vi "BM_Detect_Integrate_Peaks.vi"(8 "stop":bool, 9 "Use as SubVI?":bool, 10 "Drop\npt.s?":i32=1, 11 "Imported Data":dbl[][](array[numeric])=array14000x8[112000 elements]) -> (2 "Peak Area":dbl=9488.210393014257 format="%#_4e", 3 "Peak Height":dbl=499.997845207867 format="%#_4e")   [LabVIEW 2021]
uses:
  <vilib>/Analysis/6fits.llb/Curve Fitting Criteria.ctl
  <vilib>/Utility/miscctls.llb/LVAnnotationListTypeDef.ctl
  <vilib>/Analysis/NI_AALPro.lvlib
  <vilib>/ptbypt/NI_PtbyPt.lvlib
  <vilib>/Analysis/NI_AAL_SigProc.lvlib
  <vilib>/Analysis/NI_AALBase.lvlib
panel:
  in  "Tab Control":enum32{"GUI", "Imported Raw Data"}(tab)
  in  "Reset Plots":bool
  in  "Analyte":u16(ring) items=["62 m/z", "63 m/z", "65 m/z", "68 m/z", "70 m/z"]
  out "Detection Limit":dbl=5.772939383333335 caption="LOD" format="%#_3g"
  out "Integrated Data":cluster{dbl[], dbl[]}(graph)
  out "Data":T1(graph)
  out "X Click Coordinates":dbl=462.027422648
  out "Y Click Coordinates":dbl=59.0625
  out "Closest X Data pt.":dbl=463.592079
  out "Closest Y Data pt.":dbl=59.95878535601133
  in  "Filename":path=path "C:/Users/bcamc/OneDrive/Desktop/2022_cruise_data/CIMS_Data/Brandon_CIMS_07102022_02.lvm"
  out "X Data":dbl[](array[numeric])
  out "Y Data":dbl[](array[numeric])
  in  "YData Index":i32=7
  out "Number of Points Selected":i32
  in  "XData Index":i32=6
  in  "Width":i32=6
  in  "Correct Baseline\nOrder":bool=TRUE
  in  "Apply Boxcar Filter":bool
  out "Filtered Y":dbl[](array[numeric])
  out "Baseline Corrected Y":dbl[](array[numeric])
  out "Boxcar Progress":u8(slide) scale=0.0..100.0
  in  "Autofix Y Scale":bool=TRUE
  out "Integral Y":dbl[](array[numeric])=[40.03240345107625, -9.96789609639881, -19.96819647164608, 10.03150332578528, 10.031203296894425, -29.96909656031754, 10.030604753152069, -19.96969475828041, 0.030005903961438207, -19.97029326311293, -9.970592257508663, -29.970890086087266, 10.028811265294742, 30.02851278935423, -9.97178650433171, -29.97208562617694, -19.97238259366285, 20.027319623664553, -9.972977989306159, 50.02672358284819, -19.973574669190057, 30.02612922441501, 20.025832303719383, -29.974464444298768, 20.025238980360562, 30.02494159358664, -19.97535562133391, -49.97565069453216, -9.975946577602919, -39.97624228898213, 0.023462172316150998, 0.02316582365677533, 0.022871612945145614, -19.977423409689074, -29.977718255715935, 0.021987068969757217, 10.021691586570974, -29.978601763626443, 20.02110407713249, -19.979189906491733, -29.979484695881453, 40.02022069149108, 20.01992820042487, -29.980365093871676, 20.01934081422818, 0.019046892249846792, -19.98124685394985, -9.981538482377943, 0.01816908786275917, 20.017876832728625, 50.01758474832545, 20.01729186740849, 30.017001099498053, 40.016709535071534, 20.016418140410195, 20.016126917458827, -29.984164126026975, 20.0155459640702, 30.015255262455305, 20.014964732549217, 30.01467437435368, 50.0143832263437, 30.01409417889586, 40.013804338734495, 20.013514671251755, 60.01322517741171, 70.01293489662064, 120.01264670776405, 40.012357731956456, 80.01206797091655, 80.01177838177952, 50.01148896454879, 80.01120164120061, 70.01091353088685, 90.01062559133166, 130.0103378234968, 170.01004927444615, 140.00976280969502, 190.00947556372347, 140.00918848755913, 190.00890158502887, 250.00861485326635, 270.0083292484607, 200.00804286338996, 260.0077566519498, 290.0074706112809, 310.00718379607423, 260.0068990498817, 250.0066135291492, 290.006328181093, 310.00604300191446, 250.00575799826413, 400.0054722225604, 270.0051885099438, 440.00490402432536, 350.0046197113844, 360.00433557017465, 290.00405065977725, 470.00376780768124, 350.0034841854507, 280.0032007368416, 380.0029165185042, 420.00263247493706, 310.00235048204814, 410.002067725663, 440.00178514007087, 290.00150272621573, 370.00122048691907, 320.0009393568023, 410.00065746040724, 300.00037480133426, 410.00009231702643, 379.9998100065449, 399.9995297371525, 429.9992487062318, 459.9989678470532, 359.9986862295762, 319.9984047849914, 439.99812537762523, 499.997845207867, 389.9975642849034, 369.9972844638737, 329.99700388798567, 239.99672534077752, 279.9964460377797, 339.9961669074594, 439.99588794981656, 309.99560823832314, 369.9953305516355, 329.995052112953, 419.9947738450934, 369.9944957499124, 349.9942178292611, 419.99394100252186, 359.99366342572597, 159.9933851005939, 199.99310694836495, 229.9928289718088, 179.99255300488858, 329.9922762926282, 249.9919997539662, 369.9917224676506, 229.991445357923, 169.99117025485873, 219.99089440564006, 199.99061873093612, 269.990343227991, 179.99006698268045, 209.98979274013325, 209.98951775338915, 189.9892429420703, 79.98896830159859, 179.9886938319775, 119.98842045120503, 69.9881463300203, 249.98787237877505, 139.9875986029447, 149.98732499979067, 109.98705065967226, 139.98677827602253, 139.986505222749, 209.98623140329462, 49.9859577558501, 129.9856842840496, 179.9854127957304, 69.98514057423267, 79.98486762127854, 129.98459484396267, 119.98432223956722, 109.98405161019505, 79.98378025323284, 129.98350906894808, 119.98323805824333, 59.982966318299475, 129.98269655125742, 149.98242605858394, 119.98215573768661, 99.98188558856715, 39.98161561482343, 159.98134670683015, 169.98107707606925, 99.98080761888315, 69.9805383325799, 29.98026832458241, 39.98000027890487, 69.97973151332198, 49.97946291773094, 69.97919360274193, 99.97892446515473, 69.97865727788658, 59.97838937447513, -0.0218783562588456, 39.97785408746663, 39.97758670030564, 39.97732037477243, 89.97705333328562, 109.97678646714353, 19.97651977190037, 99.97625324844716, 89.97598778374929, 69.9757216050787, 49.975455600858375, 69.97518888496157, 49.974922343776946, 69.97465773751549, 59.974392425460934, 19.974127284315678, 59.97386143613493, 89.97359576178053, 49.97333201661638, 39.97306756763633, 89.9728032913326, 9.972539185946232, 59.97227437608945, -30.02798850503394, 29.971747907614443, 79.97148449469582, 79.9712212527003, 89.97095818338343, 9.970696161327204, -0.02956656145727976, 19.97017088756025, 79.96990850838154, 79.9696463027546, 29.969383399841476, 39.969122410405184, 19.968860721938682, -10.031400792978324, 69.96833699624216, 29.968074959290135, 19.967814830074538, -10.032445993557914, 49.96729248924528, -0.03296885238920311, 29.966769978067866, 39.96651071138221, 9.966250752284147, 49.965990965863554, 129.96573048846227, -10.034529811654537, 59.965211780157794, 19.96495268674736, 29.964693763425437, 49.96443501450545, -20.03582356259929, 29.96391889088816, -0.03633934229502245, 39.963402598919124, 19.96314471109205, 19.962886139464665, 89.96262945433142, -10.037627913746242, 39.96211488999596, 19.961857865559736, 9.961600162759488, 69.96134433728743, -0.03891216826045252, 29.96083064698272, 29.960573636053397, 9.960316799804033, 19.960061835996257, -0.040193805016087936, 79.95955072579832, -40.04070456900835, 9.959039460147565, 59.95878535601133]
  in  "polynomial order":i32=2
  in  "Threshold":dbl=650.0 format="%0.2f"
  in  "Width":i32=25 min=3
  out "Peaks\nFound":i32
  in  "Auto Detect Peaks":bool=TRUE
  out "n Blanks":i32
  in  "Calculate LOD":bool caption="2. Add Std. Peak"
  in  "Add Next Blank":bool caption="1. Add Blank Peaks (³3)"
  in  "Std. Conc.":dbl
  out "Peak Start Time":string="00:06:24"
  out "Peak Height Time":string="00:06:60"
  in  "Imported Data Table":string[][](table)=array14000x8[112000 elements]
  out "Peak \nLocations (mins)":dbl[](array[numeric])
  out "Peak \nAmplitudes":dbl[](array[numeric])
  out "Retention\nTime (min)":dbl[](array[numeric])
  out "Mean Retention Time (Min)":dbl format="%#_3g"
  # "Find and Integrate Peaks"
  # "Select Data"
  # "Selected Data Points"
  # "Integrated Peak"
  # "nM"
  # "nM"
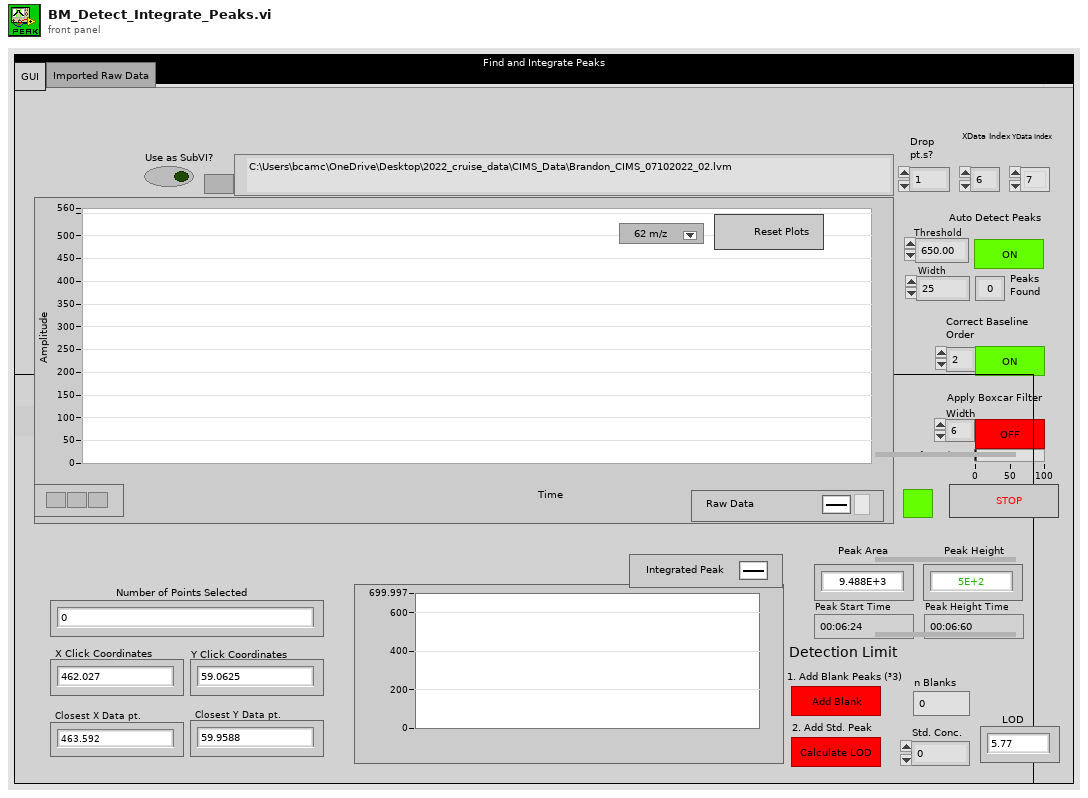
[diagram p1: front panel]
types:
  T1 = cluster{"Integral X Data":dbl[], "Integral Y Data":dbl[]}[]
  T2 = typedef "LVAnnotationListTypeDef.ctl" = cluster{"Name":string, "Color":u32, "Style":u8, "Point Style":u8, "Name Visible":bool, "Allow Drag":bool, "Annotation Mode":u32, "Plot":i32, "Index":i32, "Position":cluster{"X":dbl, "Y":dbl}, "X Scale":u32, "Y Scale":u32, "Show Arrow":bool, "Lock Name":bool, "Plot Area":i32, "Label Offset":cluster{"X":dbl, "Y":dbl}}[]
  T3 = typedef "NI_AALPro.lvlib/Curve Fitting Criteria.ctl" = u16
  T4 = cluster{"Integral X Data":dbl[], "Integral Y Data":dbl[]}
  T5 = cluster{"Name":string, "Color":u32, "Style":u8, "Point Style":u8, "Name Visible":bool, "Allow Drag":bool, "Annotation Mode":u32, "Plot":i32, "Index":i32, "Position":cluster{"X":dbl, "Y":dbl}, "X Scale":u32, "Y Scale":u32, "Show Arrow":bool, "Lock Name":bool, "Plot Area":i32, "Label Offset":cluster{"X":dbl, "Y":dbl}}
  T6 = cluster{"X Data":dbl[], "Baseline Corrected Y":dbl[]}
  T7 = typedef "LVPoint32TypeDef.ctl" = cluster{"Horizontal":i32, "Vertical":i32}
  T8 = typedef "LVRectTypeDef.ctl" = cluster{"Left":i16, "Top":i16, "Right":i16, "Bottom":i16}
  T9 = cluster{string, u32, i32, i32, bool, bool, i32, i32, i32, cluster{dbl, dbl}}
  T10 = cluster{string, u32, i32, i32, bool, bool, i32, i32, i32, cluster{dbl, dbl}}[]
  T11 = cluster{"Name":string, "Color":u32, "Style":u8, "Point Style":u8, "Name Visible":bool, "Allow Drag":bool, "Annotation Mode":u32, "Plot":i32, "Index":i32, "Position":cluster{"X":dbl, "Y":dbl}, "X Scale":u32, "Y Scale":u32, "Show Arrow":bool, "Lock Name":bool, "Plot Area":i32, "Label Offset":cluster{"X":dbl, "Y":dbl}}[]
  T12 = cluster{"X Data":dbl[], "Baseline Corrected Y":dbl[]}[]
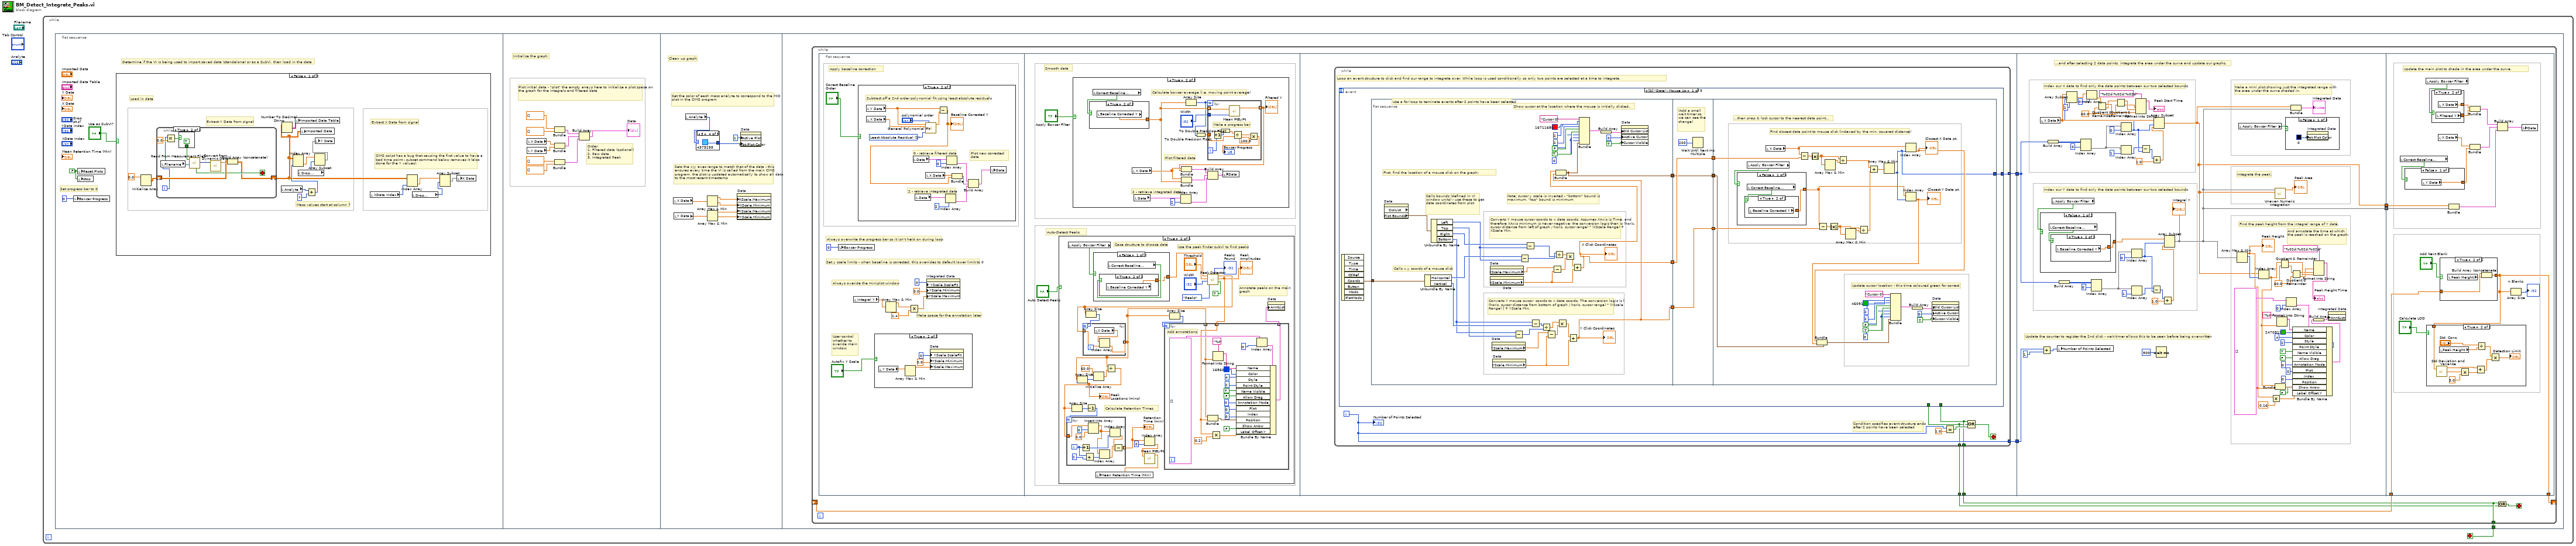
[diagram p0: block diagram]
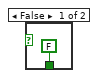
[diagram p2: hidden frame]
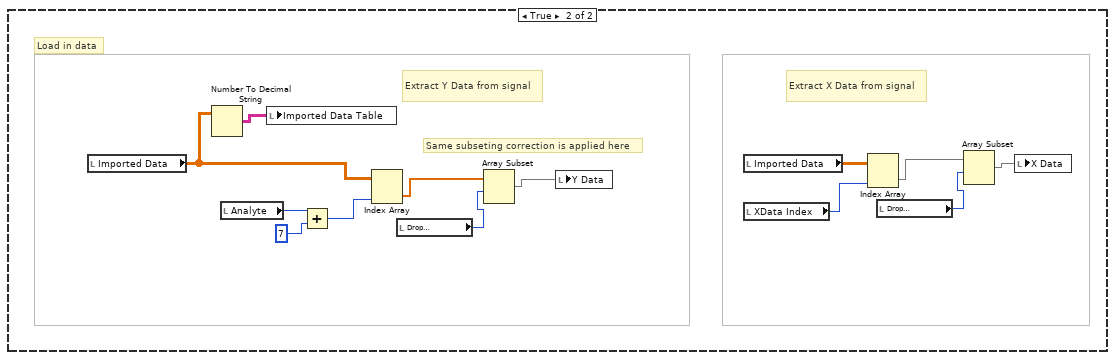
[diagram p3: hidden frame]
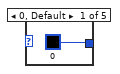
[diagram p4: hidden frame]
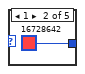
[diagram p5: hidden frame]
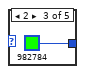
[diagram p6: hidden frame]
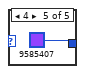
[diagram p7: hidden frame]
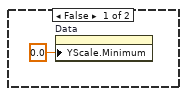
[diagram p8: hidden frame]
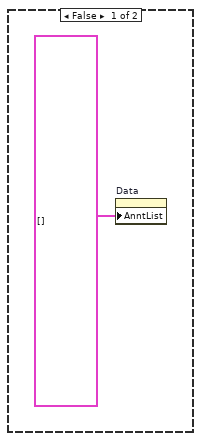
[diagram p10: hidden frame]
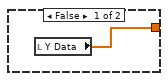
[diagram p11: hidden frame]
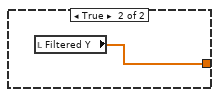
[diagram p12: hidden frame]
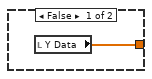
[diagram p14: hidden frame]
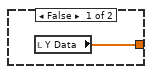
[diagram p15: hidden frame]
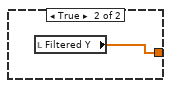
[diagram p16: hidden frame]
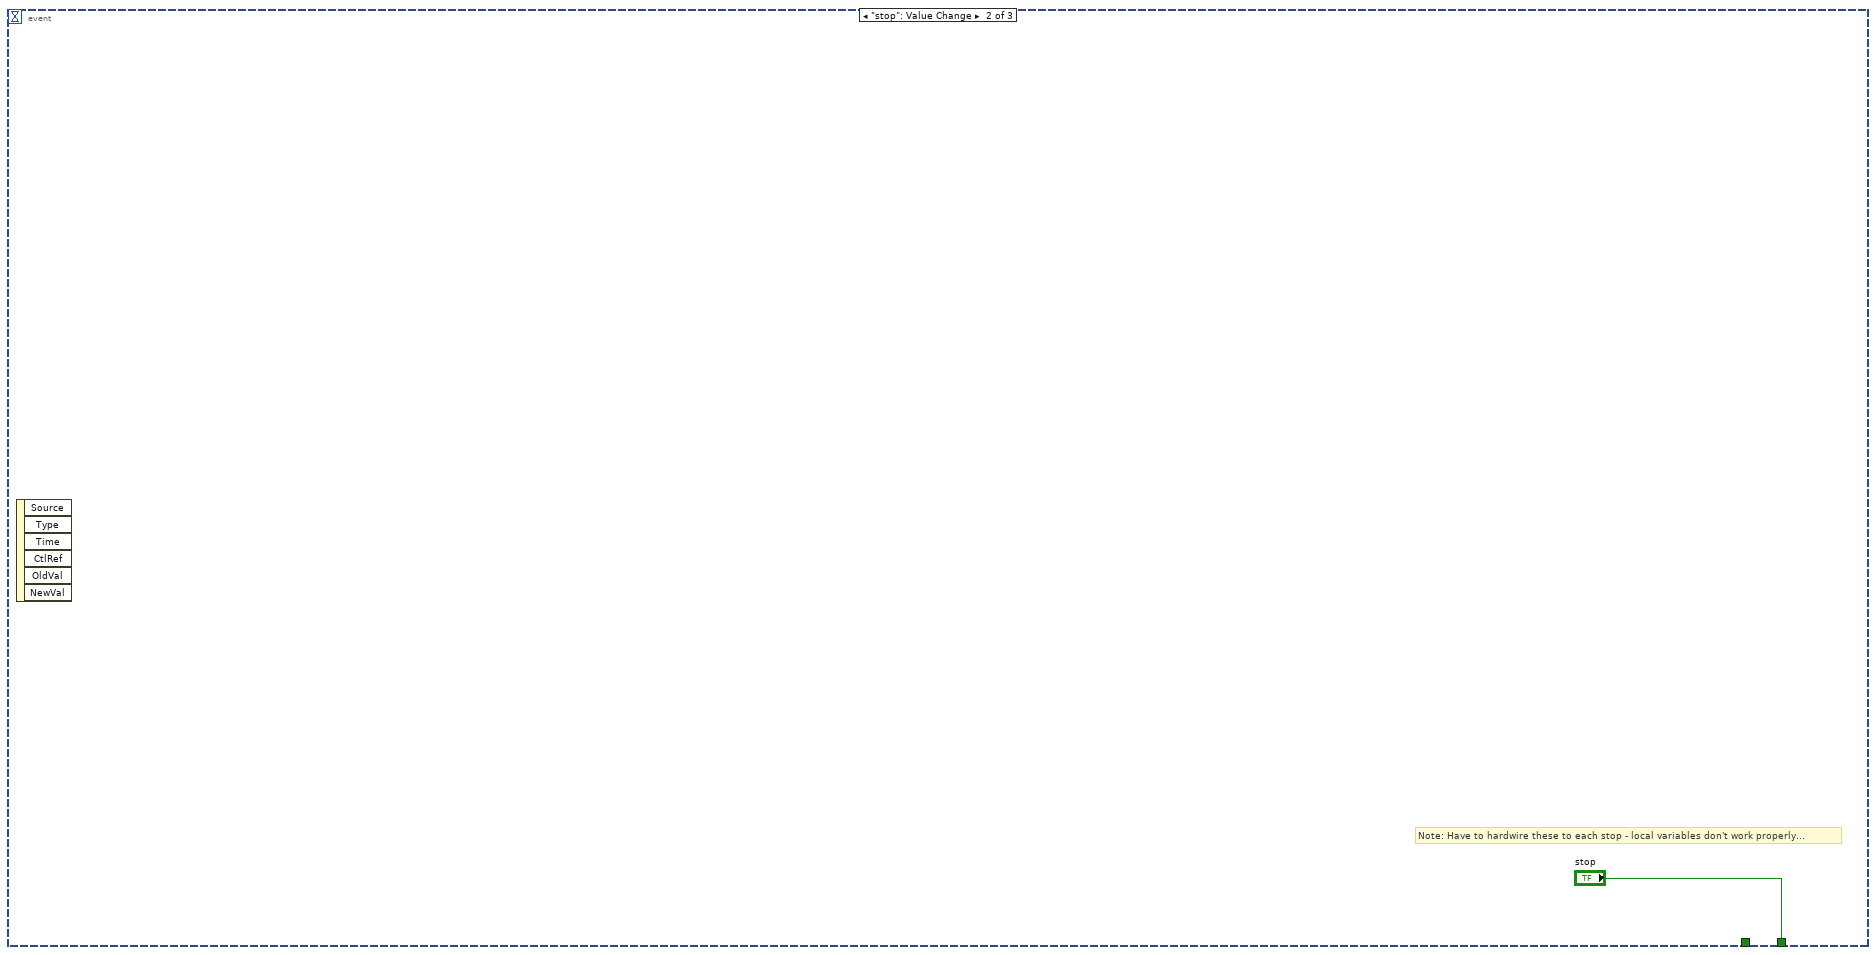
[diagram p17: hidden frame]
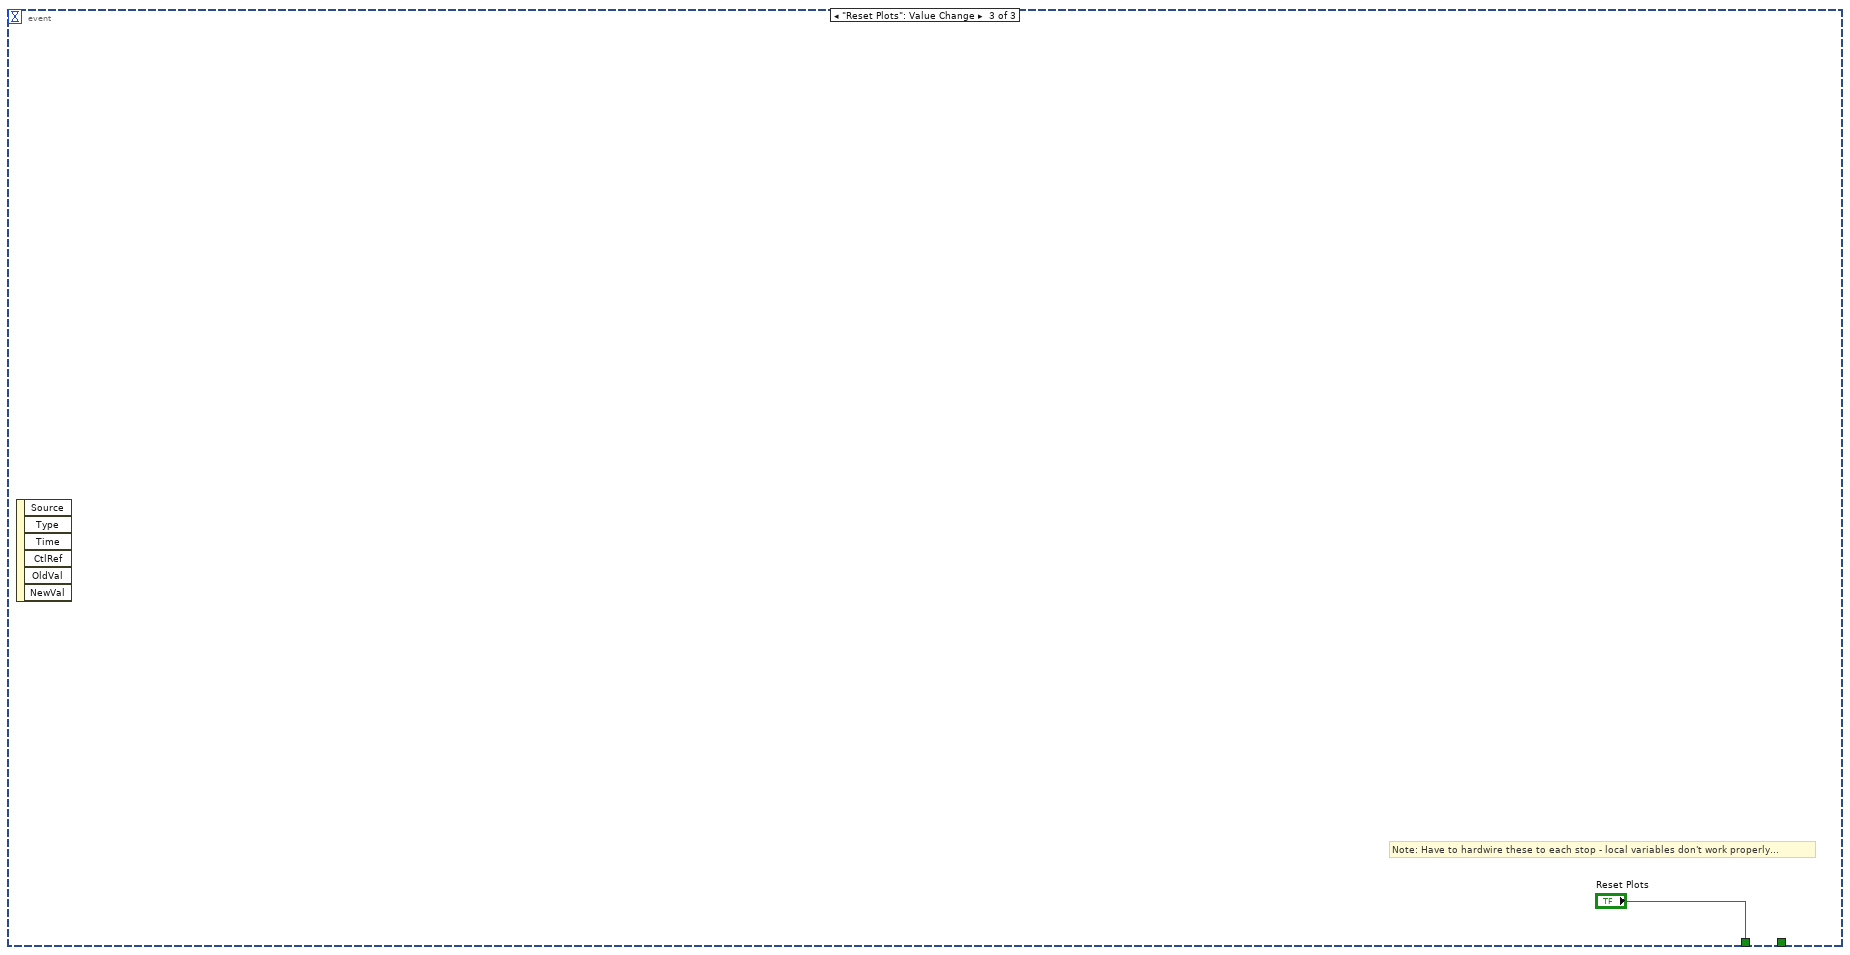
[diagram p18: hidden frame]
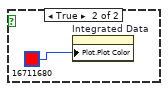
[diagram p19: hidden frame]
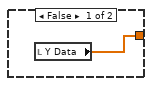
[diagram p20: hidden frame]
diagram:
  n1 = while {
    stop <- w1 stop-if-true
    n2 = flat-sequence {
      tunnel: [w68] -> w1
      frame #0 {
        w2 = FALSE ("Reset Plots")
        # "Set progress bar to 0"
        # "Determine if the VI is being used to import saved data (standalone) or as a SubVi, then load in the data"
        n3 = local write "Boxcar Progress"(u8 0 ("Boxcar Progress")) -> ()
        n4 = local write "Reset Plots"(w2) -> ()
        n5 = local write "stop"(w2) -> ()
        n6 = case shown="False" "Use as SubVI?" {
          frame False {
            # "Mass values start at column 7"
            # "CIMS script has a bug that causing the first value to have a bad time point - subset command below removes it (also done for the Y values)."
            # "Load in data"
            # "Extract X Data from signal"
            # "Extract Y Data from signal"
            n7 = Initialize Array(0.0 ("element")) -> (w7:dbl[][])  [unwired: 2 in]
            n8 = while {
              shift-right: [w25] -> w10
              shift-left: w7 -> [w27]
              i -> [w21]
              stop <- w26 stop-if-true
              n9 = local read "Filename"() -> (w19:path)
              n10 = Equal?(x=w21, y=0.0) -> (x = y?=w23:bool)
              n11 = case shown="True" w23 {
                tunnel: [FALSE TRUE] -> w20
                frame False {
                }
                frame True {
                }
              }
              n12 = call "Read From Measurement File2"("Filename"=w19, "Reset"=w20) -> ("Signals"=w24:dynamicdata, "EOF?"=w26:bool)  [unwired: 4 in, 4 out]
              n13 = call "Convert from Dynamic Data"("Dynamic Data Type"=w24) -> ("Array"=w28:dbl[])  [unwired: 3 in]
              n14 = Build Array (concatenate)(w27, w28) -> (w25:dbl[][])
            }
            n15 = local read "Analyte"() -> (w18:u16)
            n16 = Number To Decimal String(number=w10) -> (decimal integer string=w9:string[][])  [unwired: 1 in]
            n17 = local write "Imported Data Table"(w9) -> ()
            n18 = local read "Drop\npt.s?"() -> (w11:i32)
            n19 = local write "Imported Data"(w10) -> ()
            n20 = Add(x=w18, y=u16 7) -> (x+y=w17:u16)
            n21 = Index Array(array=w10, index (col)=w17) -> (element=w12:dbl[])  [unwired: 1 in]
            n22 = Array Subset(array=w12, index=w11) -> (w13:dbl[])  [unwired: 1 in]
            n23 = local write "Y Data"(w13) -> ()
            n24 = local read "XData Index"() -> (w8:i32)
            n25 = Index Array(array=w10, index (col)=w8) -> (element=w15:dbl[])  [unwired: 1 in]
            n26 = local read "Drop\npt.s?"() -> (w14:i32)
            n27 = Array Subset(array=w15, index=w14) -> (w16:dbl[])  [unwired: 1 in]
            n28 = local write "X Data"(w16) -> ()
          }
          frame True {
            # "Same subseting correction is applied here"
            # "Load in data"
            # "Extract X Data from signal"
            # "Extract Y Data from signal"
            n29 = local read "Imported Data"() -> (w35:dbl[][])
            n30 = Number To Decimal String(number=w35) -> (decimal integer string=w34:string[][])  [unwired: 1 in]
            n31 = local read "Analyte"() -> (w33:u16)
            n32 = local write "Imported Data Table"(w34) -> ()
            n33 = Add(x=w33, y=u16 7) -> (x+y=w31:u16)
            n34 = Index Array(array=w35, index (col)=w31) -> (element=w40:dbl[])  [unwired: 1 in]
            n35 = local read "Drop\npt.s?"() -> (w41:i32)
            n36 = Array Subset(array=w40, index=w41) -> (w39:dbl[])  [unwired: 1 in]
            n37 = local write "Y Data"(w39) -> ()
            n38 = local read "Imported Data"() -> (w42:dbl[][])
            n39 = local read "XData Index"() -> (w43:i32)
            n40 = Index Array(array=w42, index (col)=w43) -> (element=w37:dbl[])  [unwired: 1 in]
            n41 = local read "Drop\npt.s?"() -> (w38:i32)
            n42 = Array Subset(array=w37, index=w38) -> (w36:dbl[])  [unwired: 1 in]
            n43 = local write "X Data"(w36) -> ()
          }
        }
      }
      frame #1 {
        # "Order:\n1. Filtered data (optional)\n2. Raw data\n3. Integrated Peak"
        # "Initialize the graph"
        # "Plot initial data - \"plot\" the empty arrays here to initialize a plot space on the graph for the integrals and filtered data"
        n44 = local read "X Data"() -> (w53:dbl[])
        n45 = local read "Y Data"() -> (w52:dbl[])
        n46 = Bundle(dbl[] [], dbl[] []) -> (w45:cluster{dbl[], dbl[]})  [unwired: 1 in]
        n47 = Bundle("X Data"=w53, "Y Data"=w52) -> (w49:cluster{"X Data":dbl[], "Y Data":dbl[]})  [unwired: 1 in]
        n48 = Bundle(dbl[] [], dbl[] []) -> (w48:cluster{dbl[], dbl[]})  [unwired: 1 in]
        n49 = Build Array(w45, w49, w48) -> (→"Data":cluster{"X Data":dbl[], "Y Data":dbl[]}[])
      }
      frame #2 {
        # "Clean up graph"
        # "Sets the x/y axes range to match that of the data - this ensures every time the VI is called from the main CIMS program, the plot is updated automatically to show all data to the most recent timestamp"
        # "Set the color of each mass analyte to correspond to the MID plot in the CIMS program"
        n50 = local read "X Data"() -> (w57:dbl[])
        n51 = local read "Y Data"() -> (w56:dbl[])
        n52 = local read "Analyte"() -> (w62:u16)
        n53 = case shown="3" w62 {
          tunnel: [u32 0 ("Plot.Fill/Point Color") u32 16728642 ("Plot.Fill/Point Color") u32 982784 ("Plot.Fill/Point Color") u32 4375295 ("Plot.Fill/Point Color") u32 9585407 ("Plot.Fill/Point Color")] -> w60
          frame 0, Default {
          }
          frame 1 {
          }
          frame 2 {
          }
          frame 3 {
          }
          frame 4 {
          }
        }
        n54 = Array Max & Min(array=w57) -> (max value=w59:dbl, min value=w58:dbl)  [unwired: 2 out]
        n55 = Array Max & Min(array=w56) -> (max value=w55:dbl, min value=w54:dbl)  [unwired: 2 out]
        n56 = property on="Data" class="XYGraph (strict)"("XScale.Maximum"=w59, "XScale.Minimum"=w58, "YScale.Maximum"=w55, "YScale.Minimum"=w54) -> ()  [unwired: 2 in, 2 out]
        n57 = property on="Data" class="XYGraph (strict)"("Active Plot"=u32 1, "Plot.Plot Color"=w60) -> ()  [unwired: 2 in, 2 out]
      }
      frame #3 {
        n58 = while {
          shift-right: [w71] -> _
          shift-left: _ -> [w73]
          tunnel: [w70] -> w68
          stop <- w72 stop-if-true
          n59 = flat-sequence {
            tunnel: [w200] -> w75
            tunnel: [w199] -> w74
            tunnel: [w198] -> w70
            tunnel: [w197] -> w69
            tunnel: [w345] -> w77
            tunnel: [w314] -> w76
            tunnel: w75 -> [w346]
            tunnel: w74 -> [w343]
            tunnel: w77 -> [w384]
            tunnel: w76 -> [w385]
            tunnel: w73 -> [w377]
            tunnel: [w373] -> w71
            frame #0 {
              # "Make space for the annotation later"
              # "User control whether to overide main window"
              # "Always overide the miniplot window"
              # "Set y scale limits - when baseline is corrected, this overrides to default lower limit to 0"
              # "Always overwrite the progress bar so it isn't held on during loop"
              # "Apply baseline correction"
              n60 = local write "Boxcar Progress"(u8 0 ("Boxcar Progress")) -> ()
              n61 = local read "Integral Y"() -> (w82:dbl[])
              n62 = case shown="True" "Correct Baseline\nOrder" {
                frame False {
                }
                frame True {
                  w105 = T3 1 items=["Least Square", "Least Absolute Residual", "Bisquare"] ("method")
                  # "0 - retrieve filtered data"
                  # "2 - retrieve integrated data"
                  # "Plot new corrected data"
                  # "Subtract off a 2nd order polynomial fit using least absolute residuals"
                  n63 = local read "Y Data"() -> (w102:dbl[])
                  n64 = local read "X Data"() -> (w104:dbl[])
                  n65 = local read "Data"() -> (w94:T1)
                  n66 = local read "Data"() -> (w97:T1)
                  n67 = call <vilib>:"General Polynomial Fit.vi"("Y"=w102, "polynomial order"="polynomial order", "X"=w104, "method"=w105) -> ("Best Polynomial Fit"=w103:dbl[])  [unwired: 8 in, 3 out]
                  n68 = local read "X Data"() -> (w101:dbl[])
                  n69 = Subtract(x=w102, y=w103) -> (x-y=w100:dbl[])
                  "Baseline Corrected Y" <- w100
                  n70 = Index Array(array=w97, index=2) -> (element=w95:T4)
                  n71 = Index Array(array=w94, index=0) -> (element=w92:T4)
                  n72 = Bundle("X Data"=w101, w100) -> (w99:cluster{"X Data":dbl[], dbl[]})  [unwired: 1 in]
                  n73 = Build Array(w92, w99, w95) -> (w98:T1)
                  n74 = local write "Data"(w98) -> ()
                }
              }
              n75 = case shown="True" "Autofix Y Scale" {
                frame False {
                  n76 = property on="Data" class="XYGraph (strict)"("YScale.Minimum"=0.0 ("Y Scale.Range:Minimum")) -> ()  [unwired: 2 in, 2 out]
                }
                frame True {
                  n77 = local read "Y Data"() -> (w89:dbl[])
                  n78 = Array Max & Min(array=w89) -> (max value=w88:dbl)  [unwired: 3 out]
                  n79 = property on="Data" class="XYGraph (strict)"("YScale.ScaleFit"=u8 0 ("Y Scale.Scale Fit"), "YScale.Minimum"=0.0 ("Y Scale.Range:Minimum"), "YScale.Maximum"=w88) -> ()  [unwired: 2 in, 2 out]
                }
              }
              n80 = Array Max & Min(array=w82) -> (max value=w80:dbl)  [unwired: 3 out]
              n81 = Multiply(x=w80, y=1.4) -> (x*y=w79:dbl)
              n82 = property on="Integrated Data" class="XYGraph (strict)"("YScale.ScaleFit"=u8 0 ("Y Scale.Scale Fit"), "YScale.Minimum"=0.0 ("Y Scale.Range:Minimum"), "YScale.Maximum"=w79) -> ()  [unwired: 2 in, 2 out]
            }
            frame #1 {
              # "Auto-Detect Peaks"
              # "Smooth data"
              n83 = case shown="True" "Auto Detect Peaks" {
                frame False {
                  n84 = property on="Data" class="XYGraph (strict)"("AnntList"=T2 [] ("Annotation List")) -> ()  [unwired: 2 in, 2 out]
                }
                frame True {
                  # "Case structure to choose data"
                  # "Annotate peaks on the main graph"
                  # "Use the peak finder subVi to find peaks"
                  # "Calculate Retention Times"
                  n85 = local read "Apply Boxcar Filter"() -> (w127:bool)
                  n86 = case shown="False" w127 {
                    tunnel: [w167 w171] -> w125
                    frame False {
                      n87 = local read "Correct Baseline\nOrder"() -> (w168:bool)
                      n88 = case shown="True" w168 {
                        tunnel: [w169 w170] -> w167
                        frame False {
                          n89 = local read "Y Data"() -> (w169:dbl[])
                        }
                        frame True {
                          n90 = local read "Baseline Corrected Y"() -> (w170:dbl[])
                        }
                      }
                    }
                    frame True {
                      n91 = local read "Filtered Y"() -> (w171:dbl[])
                    }
                  }
                  n92 = call <vilib>:"Peak Detector.vi"("initialize (T)"=TRUE, "peaks/valleys"=enum32{"Peaks", "Valleys"}."Peaks", "width"="Width", "threshold"="Threshold", "X"=w125) -> ("Amplitudes"=w119:dbl[], "Locations"=w124:dbl[], "# found"=→"Peaks\nFound":i32)  [unwired: 2 in, 2 out]
                  "Peak \nAmplitudes" <- w119
                  n93 = Array Size(array=w124) -> (size(s)=w126:i32)
                  n94 = for {
                    N: w126 -> [_]
                    tunnel: w124 -> [w166] mode=indexing
                    tunnel: [w165] -> w117 mode=indexing
                    n95 = local read "X Data"() -> (w164:dbl[])
                    n96 = Index Array(array=w164, index=w166) -> (element=w165:dbl)
                  }
                  n97 = Array Size(array=w117) -> (size(s)=w123:i32)
                  n98 = Initialize Array(60.0 ("element"), w123) -> (w121:dbl[])
                  n99 = Divide(x=w117, y=w121) -> (x/y=w116:dbl[])
                  "Peak \nLocations (mins)" <- w116
                  n100 = Array Size(array=w116) -> (size(s)=w115:i32)
                  n101 = Decrement(x=w115) -> (x-1=w114:i32)
                  n102 = for {
                    N: w114 -> [_]
                    tunnel: w116 -> [w143]
                    tunnel: [w133] -> w113 mode=indexing
                    i -> [w138]
                    n103 = Increment(x=w138) -> (x+1=w137:i32)
                    n104 = Add(x=w138, y=2) -> (x+y=w140:i32)
                    n105 = Insert Into Array(array=w143, index=0, new element=0.0 ("new element/subarray")) -> (w136:dbl[])
                    n106 = Index Array(array=w136, index=w140) -> (element=w135:dbl)
                    n107 = Index Array(array=w136, index=w137) -> (element=w134:dbl)
                    n108 = Subtract(x=w135, y=w134) -> (x-y=w133:dbl)
                  }
                  "Retention\nTime (min)" <- w113
                  n109 = Index Array(array=w113, index=0) -> (element=w111:dbl)
                  n110 = call <vilib>:"Mean PtByPt.vi"("x"=w111) -> ("mean"=w110:dbl)  [unwired: 3 in, 1 out]
                  n111 = local write "Mean Retention Time (Min)"(w110) -> ()
                  n112 = Array Size(array=w117) -> (size(s)=w120:i32)
                  n113 = for {
                    N: w120 -> [_]
                    tunnel: w117 -> [w144] mode=indexing
                    tunnel: w119 -> [w152] mode=indexing
                    tunnel: [w145] -> w118 mode=indexing
                    # "Add annotations"
                    n114 = Bundle("Xo"=w144, w152) -> (w153:cluster{"Xo":dbl, dbl})  [unwired: 1 in]
                    n115 = Multiply(x=w152, y=0.2) -> (x*y=w154:dbl)
                    n116 = Format Into String(format string="%t" ("initial string"), w144) -> (resulting string=w159:string)  [unwired: 2 in, 1 out]
                    n117 = Index Array(array=T2 [] ("Annotation List"), index=0) -> (element=w161:T5)
                    n118 = Bundle By Name(cluster=w161, "Name"=w159, "Color"=u32 16860, "Style"=u8 4, "Point Style"=u8 2, "Name Visible"=TRUE, "Allow Drag"=FALSE, "Annotation Mode"=0 ("Plot"), "Plot"=0, "Index"=0, "Position"=w153, "Show Arrow"=FALSE, "Label Offset.Y"=w154) -> (w145:T5)
                  }
                  n119 = property on="Data" class="XYGraph (strict)"("AnntList"=w118) -> ()  [unwired: 2 in, 2 out]
                }
              }
              n120 = case shown="True" "Apply Boxcar Filter" {
                frame False {
                }
                frame True {
                  # "2 - retrieve integrated data"
                  # "Calculate boxcar average (i.e. moving point average)"
                  # "Plot filtered data"
                  n121 = local read "Correct Baseline\nOrder"() -> (w179:bool)
                  n122 = case shown="True" w179 {
                    tunnel: [w185 w186] -> w178
                    frame False {
                      n123 = local read "Y Data"() -> (w185:dbl[])
                    }
                    frame True {
                      n124 = local read "Baseline Corrected Y"() -> (w186:dbl[])
                    }
                  }
                  n125 = local read "X Data"() -> (w184:dbl[])
                  n126 = local read "Data"() -> (w174:T1)
                  n127 = Index Array(array=w174, index=2) -> (element=w172:T4)
                  n128 = Bundle("X Data"=w184, "Baseline Corrected Y"=w178) -> (w182:T6)  [unwired: 1 in]
                  n129 = Array Size(array=w178) -> (size(s)=w175:i32)
                  n130 = To Double Precision Float(number=w175) -> (double precision float=w176:dbl)
                  n131 = for {
                    N: w175 -> [_]
                    tunnel: w178 -> [w196] mode=indexing
                    tunnel: [w195] -> w180 mode=indexing
                    tunnel: "Width" -> [w194]
                    tunnel: w176 -> [w191]
                    i -> [w190]
                    # "Make a progress bar"
                    n132 = Increment(x=w190) -> (x+1=w189:i32)
                    n133 = To Double Precision Float(number=w189) -> (double precision float=w188:dbl)
                    n134 = call <vilib>:"Mean PtByPt.vi"("x"=w196, "sample length"=w194) -> ("mean"=w195:dbl)  [unwired: 2 in, 1 out]
                    n135 = Divide(x=w188, y=w191) -> (x/y=w193:dbl)
                    n136 = Multiply(x=w193, y=100.0) -> (x*y=→"Boxcar Progress":dbl)
                  }
                  "Filtered Y" <- w180
                  n137 = Bundle("X Data"=w184, w180) -> (w183:cluster{"X Data":dbl[], dbl[]})  [unwired: 1 in]
                  n138 = Build Array(w183, w182, w172) -> (w181:T1)
                  n139 = local write "Data"(w181) -> ()
                }
              }
            }
            frame #2 {
              n140 = while {
                tunnel: [w207] -> w200 mode=indexing
                tunnel: [w206] -> w199
                tunnel: [w202] -> w198
                tunnel: [w201] -> w197
                i -> [w206]
                stop <- w204 stop-if-true
                # "Loop an event structure to click and find our range to integrate over. While loop is used conditionally so only two points are selected at a time to integrate."
                # "Use a for loop to teminate events after 2 points have been selected"
                # "Condition specifies event structure ends after 2 points have been selected"
                n141 = event shown="[0] \"Data\": Mouse Up" {
                  selector: _ -> [_ _ _]
                  dyn-events: _ -> [_ _ _]
                  timeout: _ -> [_ _ _]
                  tunnel: [w208 _ _] -> w207
                  tunnel: [_ "stop" _] -> w202
                  tunnel: [_ _ "Reset Plots"] -> w201
                  event "Data": Mouse Up {
                    n142 = event-data() -> ("Coords"=w215:T7)  [unwired: 1 in, 7 out]
                    n143 = flat-sequence {
                      tunnel: [w216] -> w212
                      tunnel: [w233] -> w214
                      tunnel: [w225] -> w210
                      tunnel: w215 -> [w234]
                      tunnel: w214 -> [w255]
                      tunnel: [w255] -> w213
                      tunnel: w212 -> [w254]
                      tunnel: [w254] -> w211
                      tunnel: w210 -> [w253]
                      tunnel: [w253] -> w209
                      tunnel: w213 -> [w274]
                      tunnel: w211 -> [w285]
                      tunnel: w209 -> [w265]
                      tunnel: [w266] -> w208
                      frame #0 {
                        w226 = 0
                        # "First, find the location of a mouse click on the graph:"
                        # "Show cursor at the location where the mouse is initially clicked.."
                        # "Converts Y mouse cursor  coords to x data coords. The conversion logic is [ (horiz. cursor distance from bottom of graph / horiz. cursor range) * (YScale Range) ] + YScale Min."
                        # "Note: cursor y scale is inverted - \"bottom\" bound is maximum, \"top\" bound is minimum"
                        # "Converts Y mouse cursor coords to x data coords. Assumes XAxis is Time, and therefore XAxis minimum is never negative; the conversion logic then is (horiz. cursor distance from left of graph / horiz. cursor range) * (XScale Range) + XScale Min."
                        # "Calls x,y coords of a mouse click"
                        # "Calls bounds (defined in VI window units) - use these to get data coordinates from plot"
                        n144 = property on="Data" class="XYGraph (strict)" props=["CrsrList", "Plot Bounds"]() -> ("Plot Bounds"=w251:T8)  [unwired: 2 in, 3 out]
                        n145 = Unbundle By Name(w234) -> ("Horizontal"=w245:i32, "Vertical"=w240:i32)
                        n146 = Unbundle By Name(w251) -> ("Left"=w247:i16, "Top"=w238:i16, "Right"=w246:i16, "Bottom"=w239:i16)
                        n147 = property on="Data" class="XYGraph (strict)"() -> ("XScale.Maximum"=w220:dbl)  [unwired: 2 in, 2 out]
                        n148 = property on="Data" class="XYGraph (strict)"() -> ("XScale.Minimum"=w218:dbl)  [unwired: 2 in, 2 out]
                        n149 = property on="Data" class="XYGraph (strict)"() -> ("YScale.Maximum"=w242:dbl)  [unwired: 2 in, 2 out]
                        n150 = property on="Data" class="XYGraph (strict)"() -> ("YScale.Minimum"=w235:dbl)  [unwired: 2 in, 2 out]
                        n151 = Subtract(x=w239, y=w238) -> (x-y=w237:i16)
                        n152 = Subtract(x=w245, y=w247) -> (x-y=w249:i32)
                        n153 = Subtract(x=w246, y=w247) -> (x-y=w248:i16)
                        n154 = Subtract(x=w239, y=w240) -> (x-y=w244:i32)
                        n155 = Divide(x=w244, y=w237) -> (x/y=w243:dbl)
                        n156 = Subtract(x=w242, y=w235) -> (x-y=w241:dbl)
                        n157 = Subtract(x=w220, y=w218) -> (x-y=w219:dbl)
                        n158 = Divide(x=w249, y=w248) -> (x/y=w250:dbl)
                        n159 = Multiply(x=w243, y=w241) -> (x*y=w236:dbl)
                        n160 = Multiply(x=w250, y=w219) -> (x*y=w217:dbl)
                        n161 = Add(x=w236, y=w235) -> (x+y=w233:dbl)
                        "Y Click Coordinates" <- w233
                        n162 = Add(x=w217, y=w218) -> (x+y=w216:dbl)
                        "X Click Coordinates" <- w216
                        n163 = Bundle(w216, w233) -> (w225:cluster{dbl, dbl})  [unwired: 1 in]
                        n164 = Bundle("Cursor 0", u32 16711680, 2, 2, FALSE, TRUE, w226, w226, w226, w225) -> (w232:T9)  [unwired: 1 in]
                        n165 = Build Array(w232) -> (w223:T10)
                        n166 = property on="Data" class="XYGraph (strict)"("Old Cursor List"=w223, "Active Cursor"=u32 0, "Cursor.Visible"=TRUE) -> ()  [unwired: 2 in, 2 out]
                      }
                      frame #1 {
                        # "(Add a small wait timer so we can see the change)"
                        n167 = Wait Until Next ms Multiple(millisecond multiple=u32 200) -> ()  [unwired: 1 out]
                      }
                      frame #2 {
                        w276 = 0
                        # "Update cursor location - this time coloured green for correct"
                        # "Find closest data point to mouse click (indexed by the min. squared distance)"
                        # "...then snap & lock cursor to the nearest data point..."
                        n168 = local read "Apply Boxcar Filter"() -> (w262:bool)
                        n169 = case shown="False" w262 {
                          tunnel: [w287 w290] -> w263
                          frame False {
                            n170 = local read "Correct Baseline\nOrder"() -> (w286:bool)
                            n171 = case shown="True" w286 {
                              tunnel: [w288 w289] -> w287
                              frame False {
                                n172 = local read "Y Data"() -> (w288:dbl[])
                              }
                              frame True {
                                n173 = local read "Baseline Corrected Y"() -> (w289:dbl[])
                              }
                            }
                          }
                          frame True {
                            n174 = local read "Filtered Y"() -> (w290:dbl[])
                          }
                        }
                        n175 = local read "X Data"() -> (w264:dbl[])
                        n176 = Subtract(x=w264, y=w285) -> (x-y=w284:dbl[])
                        n177 = Absolute Value(x=w284) -> (abs(x)=w260:dbl[])
                        n178 = Subtract(x=w263, y=w274) -> (x-y=w275:dbl[])
                        n179 = Array Max & Min(array=w260) -> (max value=w261:dbl)  [unwired: 3 out]
                        n180 = Absolute Value(x=w275) -> (abs(x)=w257:dbl[])
                        n181 = Divide(x=w260, y=w261) -> (x/y=w259:dbl[])
                        n182 = Array Max & Min(array=w257) -> (max value=w258:dbl)  [unwired: 3 out]
                        n183 = Divide(x=w257, y=w258) -> (x/y=w256:dbl[])
                        n184 = Add(x=w259, y=w256) -> (x+y=w273:dbl[])
                        n185 = Array Max & Min(array=w273) -> (min index (indices)=w266:i32)  [unwired: 3 out]
                        n186 = Index Array(array=w264, index=w266) -> (element=w268:dbl)
                        "Closest X Data pt." <- w268
                        n187 = Index Array(array=w263, index=w266) -> (element=w267:dbl)
                        "Closest Y Data pt." <- w267
                        n188 = Bundle(cluster=w265, w268, w267) -> (w282:cluster{dbl, dbl})
                        n189 = Bundle("Cursor 0", u32 46091, 2, 2, FALSE, TRUE, w276, w276, w276, w282) -> (w283:T9)  [unwired: 1 in]
                        n190 = Build Array(w283) -> (w271:T10)
                        n191 = property on="Data" class="XYGraph (strict)"("Old Cursor List"=w271, "Active Cursor"=u32 0, "Cursor.Visible"=TRUE) -> ()  [unwired: 2 in, 2 out]
                      }
                    }
                  }
                  event "stop": Value Change {
                    # "Note: Have to hardwire these to each stop - local variables don't work properly..."
                    n192 = event-data() -> ()  [unwired: 1 in, 6 out]
                  }
                  event "Reset Plots": Value Change {
                    # "Note: Have to hardwire these to each stop - local variables don't work properly..."
                    n193 = event-data() -> ()  [unwired: 1 in, 6 out]
                  }
                }
                n194 = Equal?(x=w206, y=1.0) -> (x = y?=w203:bool)
                n195 = Compound Arithmetic op=OR(w202, w201, w203) -> (w204:bool)
                "Number of Points Selected" <- w206
              }
            }
            frame #3 {
              w299 = 60.0 ("y")
              w306 = 60.0 ("y")
              # "And annotate the time at which the peak is reached on the graph:"
              # "Update the counter to register the 2nd click - wait timer allows this to be seen before being overwritten"
              # "Integrate the peak."
              # "Find the peak height from the integral range of Y data."
              # "Make a mini plot showing just the integrated range with the area under the curve shaded in."
              # "Index our Y data to find only the data points between our two selected bounds"
              # "Index our X data to find only the data points between our two selected bounds"
              # "...and after selecting 2 data points, integrate the area under the curve and update our graphs."
              n196 = local read "X Data"() -> (w313:dbl[])
              n197 = Add(x=w343, y=1) -> (x+y=w341:i32)
              n198 = Build Array(w346) -> (w364:i32[][])
              n199 = local read "Apply Boxcar Filter"() -> (w339:bool)
              n200 = case shown="False" w339 {
                tunnel: [w369 w372] -> w347
                frame False {
                  n201 = local read "Correct Baseline\nOrder"() -> (w368:bool)
                  n202 = case shown="True" w368 {
                    tunnel: [w370 w371] -> w369
                    frame False {
                      n203 = local read "Y Data"() -> (w370:dbl[])
                    }
                    frame True {
                      n204 = local read "Baseline Corrected Y"() -> (w371:dbl[])
                    }
                  }
                }
                frame True {
                  n205 = local read "Filtered Y"() -> (w372:dbl[])
                }
              }
              n206 = local write "Number of Points Selected"(w341) -> ()
              n207 = Build Array(w346) -> (w356:i32[][])
              n208 = Index Array(array=w364, index (row)=0) -> (element=w362:i32[])  [unwired: 1 in]
              n209 = Index Array(array=w356, index (row)=0) -> (element=w354:i32[])  [unwired: 1 in]
              n210 = Index Array(array=w362, index=0) -> (element=w312:i32)
              n211 = Array Subset(array=w313, index=w312, length=1) -> (w309:dbl[])
              n212 = Index Array(array=w309, index=0) -> (element=w307:dbl)
              n213 = Quotient & Remainder(x=w307, y=w306) -> (x-y*floor(x/y)=w310:dbl, floor(x/y)=w305:dbl)
              n214 = Quotient & Remainder(x=w305, y=w306) -> (x-y*floor(x/y)=w304:dbl, floor(x/y)=w303:dbl)
              n215 = Index Array(array=w362, index=1) -> (element=w315:i32)
              n216 = Index Array(array=w354, index=0) -> (element=w344:i32)
              n217 = Index Array(array=w354, index=1) -> (element=w349:i32)
              n218 = Format Into String(format string="%02d:%02d:%02d", w303, w304, w310) -> (resulting string=→"Peak Start Time":string)  [unwired: 2 in, 1 out]
              n219 = Subtract(x=w315, y=w312) -> (x-y=w359:i32)
              n220 = Add(x=w359, y=1.0) -> (x+y=w357:dbl)
              n221 = Subtract(x=w349, y=w344) -> (x-y=w351:i32)
              n222 = Array Subset(array=w313, index=w312, length=w357) -> (w314:dbl[])
              n223 = Wait (ms)(milliseconds to wait=u32 500) -> ()  [unwired: 1 out]
              n224 = Add(x=w351, y=1.0) -> (x+y=w348:dbl)
              n225 = Array Subset(array=w347, index=w344, length=w348) -> (w345:dbl[])
              "Integral Y" <- w345
              n226 = Array Max & Min(array=w345) -> (max value=w318:dbl, max index (indices)=w337:i32)  [unwired: 2 out]
              "Peak Height" <- w318
              n227 = local read "Apply Boxcar Filter"() -> (w338:bool)
              n228 = Index Array(array=w314, index=w337) -> (element=w300:dbl)
              n229 = Multiply(x=w318, y=0.16) -> (x*y=w317:dbl)
              n230 = call <vilib>:"Uneven Numeric Integration.vi"("T"=w314, "X"=w345) -> ("result"=→"Peak Area":dbl)  [unwired: 8 in, 1 out]
              n231 = Bundle("Xo"=w300, w318) -> (w328:cluster{"Xo":dbl, dbl})  [unwired: 1 in]
              n232 = Format Into String(format string="%t", w300) -> (resulting string=w331:string)  [unwired: 2 in, 1 out]
              n233 = Quotient & Remainder(x=w300, y=w299) -> (x-y*floor(x/y)=w297:dbl, floor(x/y)=w298:dbl)
              n234 = case shown="False" w338 {
                frame False {
                  n235 = property on="Integrated Data" class="XYGraph (strict)"("Plot.Plot Color"=u32 0) -> ()  [unwired: 2 in, 2 out]
                }
                frame True {
                  n236 = property on="Integrated Data" class="XYGraph (strict)"("Plot.Plot Color"=u32 16711680) -> ()  [unwired: 2 in, 2 out]
                }
              }
              n237 = Index Array(array=T2 [] ("Annotation List"), index=0) -> (element=w332:T5)
              n238 = Bundle(w314, w345) -> (→"Integrated Data":cluster{dbl[], dbl[]})  [unwired: 1 in]
              n239 = Quotient & Remainder(x=w298, y=w299) -> (x-y*floor(x/y)=w296:dbl, floor(x/y)=w295:dbl)
              n240 = Bundle By Name(cluster=w332, "Name"=w331, "Color"=u32 2470912, "Style"=u8 4, "Point Style"=u8 2, "Name Visible"=TRUE, "Allow Drag"=FALSE, "Annotation Mode"=u32 0, "Plot"=0, "Index"=0, "Position"=w328, "Show Arrow"=FALSE, "Label Offset.Y"=w317) -> (w330:T5)
              n241 = Format Into String(format string="%02d:%02d:%02d", w295, w296, w297) -> (resulting string=→"Peak Height Time":string)  [unwired: 2 in, 1 out]
              n242 = Build Array(w330) -> (w329:T11)
              n243 = property on="Integrated Data" class="XYGraph (strict)"("AnntList"=w329) -> ()  [unwired: 2 in, 2 out]
            }
            frame #4 {
              # "Update the main plot to shade in the area under the curve."
              n244 = local read "Correct Baseline\nOrder"() -> (w378:bool)
              n245 = case shown="False" w378 {
                tunnel: [w404 w405] -> w379
                frame False {
                  n246 = local read "Y Data"() -> (w404:dbl[])
                }
                frame True {
                  n247 = local read "Baseline Corrected Y"() -> (w405:dbl[])
                }
              }
              n248 = local read "Apply Boxcar Filter"() -> (w383:bool)
              n249 = case shown="True" w383 {
                tunnel: [dbl[] [] w409] -> w382
                tunnel: [dbl[] [] w408] -> w381
                frame False {
                }
                frame True {
                  n250 = local read "Filtered Y"() -> (w408:dbl[])
                  n251 = local read "X Data"() -> (w409:dbl[])
                }
              }
              n252 = local read "X Data"() -> (w387:dbl[])
              n253 = case shown="True" "Add Next Blank" {
                tunnel: [w390 w392] -> w373
                tunnel: w377 -> [w390 w391]
                frame False {
                }
                frame True {
                  n254 = local read "Peak Height"() -> (w393:dbl)
                  n255 = Build Array (concatenate)(w391, w393) -> (w392:dbl[])
                }
              }
              n256 = case shown="True" "Calculate LOD" {
                tunnel: w373 -> [_ w401]
                frame False {
                }
                frame True {
                  n257 = call <vilib>:"Std Deviation and Variance.vi"("X"=w401) -> ("mean"=w400:dbl, "standard deviation"=w403:dbl)  [unwired: 1 in, 1 out]
                  n258 = local read "Peak Height"() -> (w398:dbl)
                  n259 = Multiply(x=w403, y=3.0) -> (x*y=w399:dbl)
                  n260 = Add(x=w400, y=w399) -> (x+y=w395:dbl)
                  n261 = Divide(x="Std. Conc.", y=w398) -> (x/y=w396:dbl)
                  n262 = Multiply(x=w396, y=w395) -> (x*y=→"Detection Limit":dbl)
                }
              }
              n263 = Bundle(w385, w384) -> (w388:cluster{dbl[], dbl[]})  [unwired: 1 in]
              n264 = Bundle("X Data"=w382, "Filtered Y"=w381) -> (w380:cluster{"X Data":dbl[], "Filtered Y":dbl[]})  [unwired: 1 in]
              n265 = Bundle("X Data"=w387, "Baseline Corrected Y"=w379) -> (w389:T6)  [unwired: 1 in]
              n266 = Build Array(w380, w389, w388) -> (w386:T12)
              n267 = Array Size(array=w373) -> (size(s)=→"n Blanks":i32)
              n268 = local write "Data"(w386) -> ()
            }
          }
          n269 = Or(x=w70, y=w69) -> (x .or. y?=w72:bool)
        }
      }
    }
  }
